vi "Configure Triggered Voltage Level [TRG].vi"(8 "error in (no error)":errorcluster, 9 "triggered level (0.0 Volts)":dbl[unit] format="%^.2e", 10 "channel name (\"CHANNEL1\")":string="CHANNEL1", 11 "CS++DCPwr in":refnum<class "CS++DCPwr.lvclass">) -> (0 "error out":errorcluster, 3 "CS++DCPwr out":refnum<class "CS++DCPwr.lvclass">)   [LabVIEW 2013, in "CS++DCPwr.lvlib" / "CS++DCPwr.lvclass"]
doc: "This VI configures the DC voltage level the power supply attempts to generate after it receives a trigger.\n\nNotes:\n\n(1) This VI is part of the IviDCPwrTrigger [TRG] extension group."
uses:
  CS++DCPwr.lvclass
  CSPP_Core/Classes/CS++ProcessVariables/ProcessVariable/PV.lvclass
  PV-Enum.ctl
  CSPP_Core/Classes/CS++ProcessVariables/ProcessVariable/PV.lvclass/PV.ctl
  CS++DCPwr.lvclass/CS++DCPwr.ctl
  CSPP_Core/Classes/CS++ProcessVariables/PVConnection/PVConnection.lvclass
  CSPP_Core/Classes/CS++ProcessVariables/ProcessVariable/Write Data.vi
  CSPP_Core/Classes/CS++ProcessVariables/ProcessVariable/Write Timestamp.vi
  CSPP_Core/Classes/CS++ProcessVariables/ProcessVariable/Write Quality.vi
  CSPP_Core/Classes/CS++ProcessVariables/ProcessVariable/Write status.vi
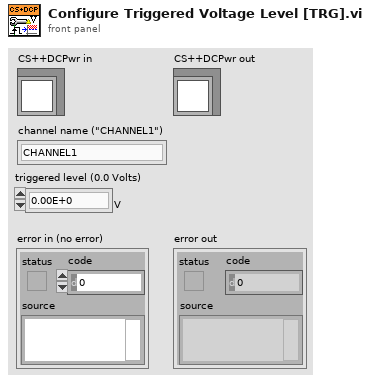
[diagram p1: front panel]
types:
  T1 = typedef "CS++DCPwr.lvlib/CS++DCPwr.lvclass/PV-Enum.ctl" = enum16{"CurrentLimit", "MaxCurrentLimit", "MaxVoltageLevel", "Measure-A", "Measure-V", "OVPLimit", "Range", "TriggerCurrentLimit", "TriggerVoltageLevel", "VoltageLevel", "Behavoir", "DesiredOutputState", "RangeType", "TriggerSource", "InState", "OutputEnable", "OVPEnabled"}
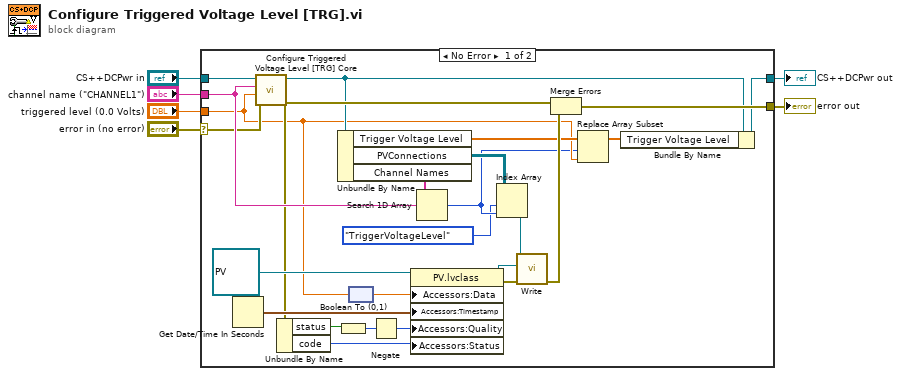
[diagram p0: block diagram]
diagram:
  n1 = case shown="No Error" "error in (no error)" {
    selector: "error in (no error)" -> [w11 w32]
    tunnel: "CS++DCPwr in" -> [w31 w33]
    tunnel: "triggered level (0.0 Volts)" -> [w10 _]
    tunnel: "channel name (\"CHANNEL1\")" -> [w18 _]
    tunnel: [w16 w32] -> w4
    tunnel: [w14 w33] -> w5
    frame No Error {
      n2 = Get Date/Time In Seconds() -> (seconds since 1Jan1904=w30:timestamp)
      n3 = call-dynamic "Configure Triggered Voltage Level [TRG] Core.vi"("error in (no error)"=w11, "triggered level (0.0 Volts)"=w10, "channel name (\"CHANNEL1\")"=w18, "CS++DCPwr in"=w31) -> ("error out"=w17:errorcluster, "CS++DCPwr out"=w15:refnum<class "CS++DCPwr.lvclass">)  [unwired: 6 in]
      n4 = Unbundle By Name(w17) -> ("status"=w22:bool, "code"=w20:i32)
      n5 = Unbundle By Name(w15) -> ("Trigger Voltage Level"=w13:dbl[unit][], "PVConnections"=w25:refnum<class "PVConnection.lvclass">[][], "Channel Names"=w26:string[])
      n6 = Boolean To (0,1)(Boolean=w22) -> (0, 1=w21:i16)
      n7 = node(w10) -> (w9:dbl)
      n8 = Negate(x=w21) -> (-x=w19:i16)
      n9 = property class="PV.lvclass"(reference=refnum<class "PV.lvclass"> refnum ("PV"), "Accessors:Data"=w9, "Accessors:Timestamp"=w30, "Accessors:Quality"=w19, "Accessors:Status"=w20) -> (reference out=w27:refnum<class "PV.lvclass">, error out=w28:errorcluster)  [unwired: 1 in]
      n10 = Search 1D Array(1D array=w26, element=w18) -> (index of element=w8:i32)  [unwired: 1 in]
      n11 = Index Array(array=w25, index (row)=PV-Enum."TriggerVoltageLevel" ("PV-Enum"), index (col)=w8) -> (element=w24:refnum<class "PVConnection.lvclass">)
      n12 = call-dynamic "Write.vi"("error in (no error)"=w28, "PV"=w27, "PVConnection in"=w24) -> ("error out"=w23:errorcluster)  [unwired: 7 in, 1 out]
      n13 = Merge Errors(w17, w23) -> (w16:errorcluster)
      n14 = Replace Array Subset(array=w13, new element=w10, index=w8) -> (w12:dbl[unit][])
      n15 = Bundle By Name(cluster=w15, "Trigger Voltage Level"=w12) -> (w14:refnum<class "CS++DCPwr.lvclass">)
    }
    frame Error {
    }
  }
  "error out" <- w4
  "CS++DCPwr out" <- w5
